vi "课堂.vi"() -> ()   [LabVIEW 2018]
panel:
  in  "停止 3":bool
  in  "等待时间（毫秒） 2":u32=1000
  out "布尔 4":bool
  out "布尔 3":bool
  out "布尔 2":bool
  out "平方根":dbl
  in  "数值":dbl
  out "数组 2":dbl[](array[numeric])
  in  "等待时间（毫秒）":u32
  in  "y 2":dbl
  in  "x 2":dbl
  in  "数组":enum16{"加法", "减法", "乘法", "除法", "清零"}[](array[ring])
  in  "停止 2":bool
  out "数值 3":dbl
  in  "y":dbl
  in  "x":dbl
  in  "枚举 2":enum16{"加法", "减法", "乘法", "除法", "清零"}(ring)
  in  "停止":bool
  out "字符串":string
  in  "枚举":enum16{"C", "B", "A"}(ring)
  out "x±1":dbl
  in  "x":dbl
  in  "布尔":bool
  # "灯亮x+1，灯灭x-1"
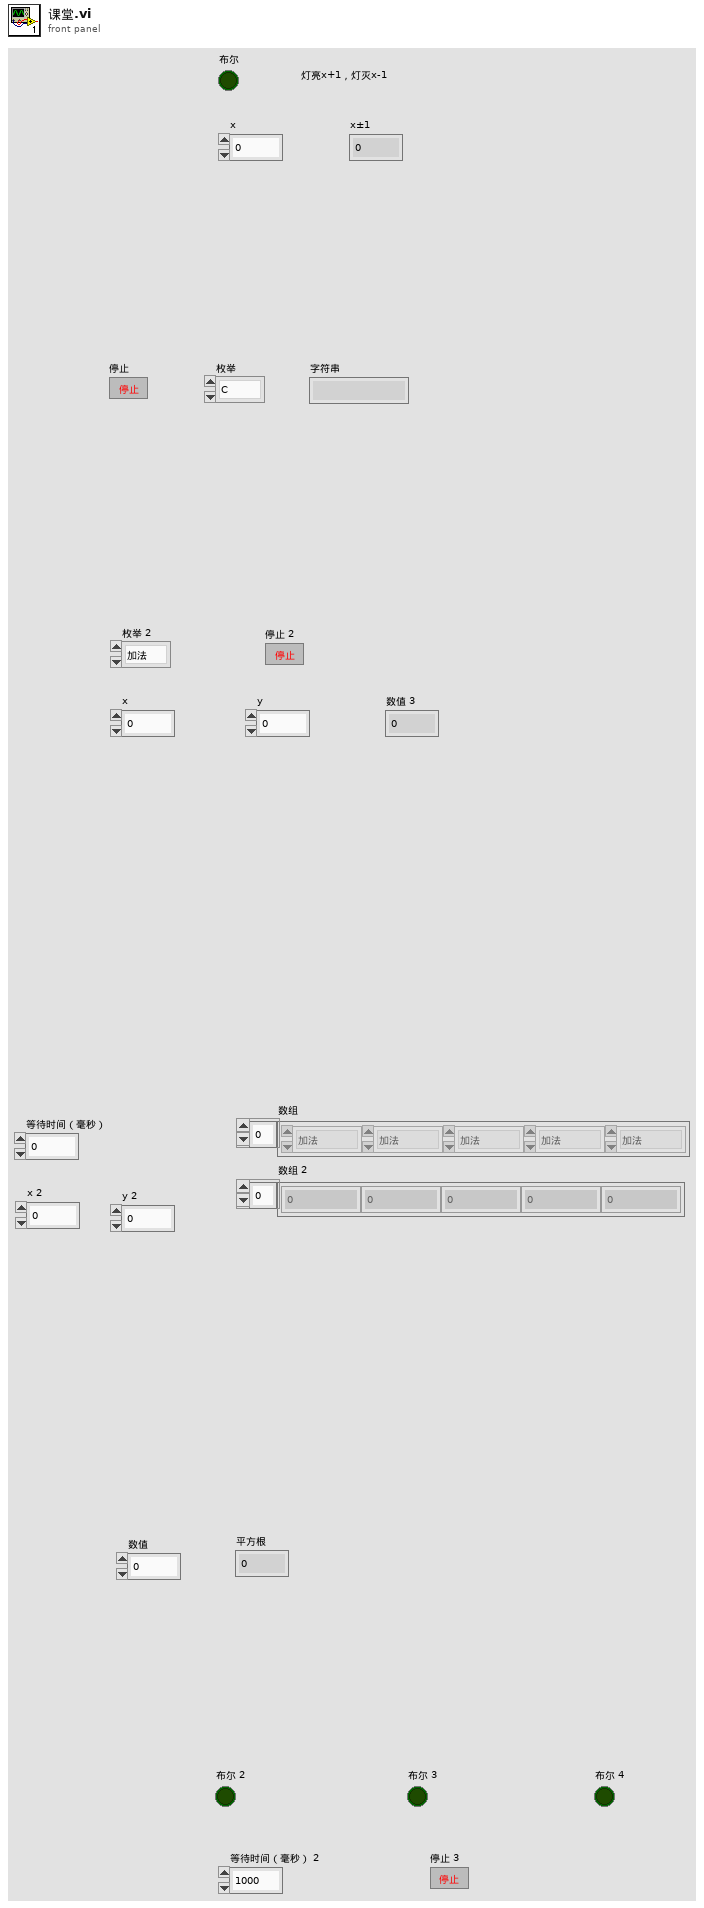
[diagram p1: front panel]
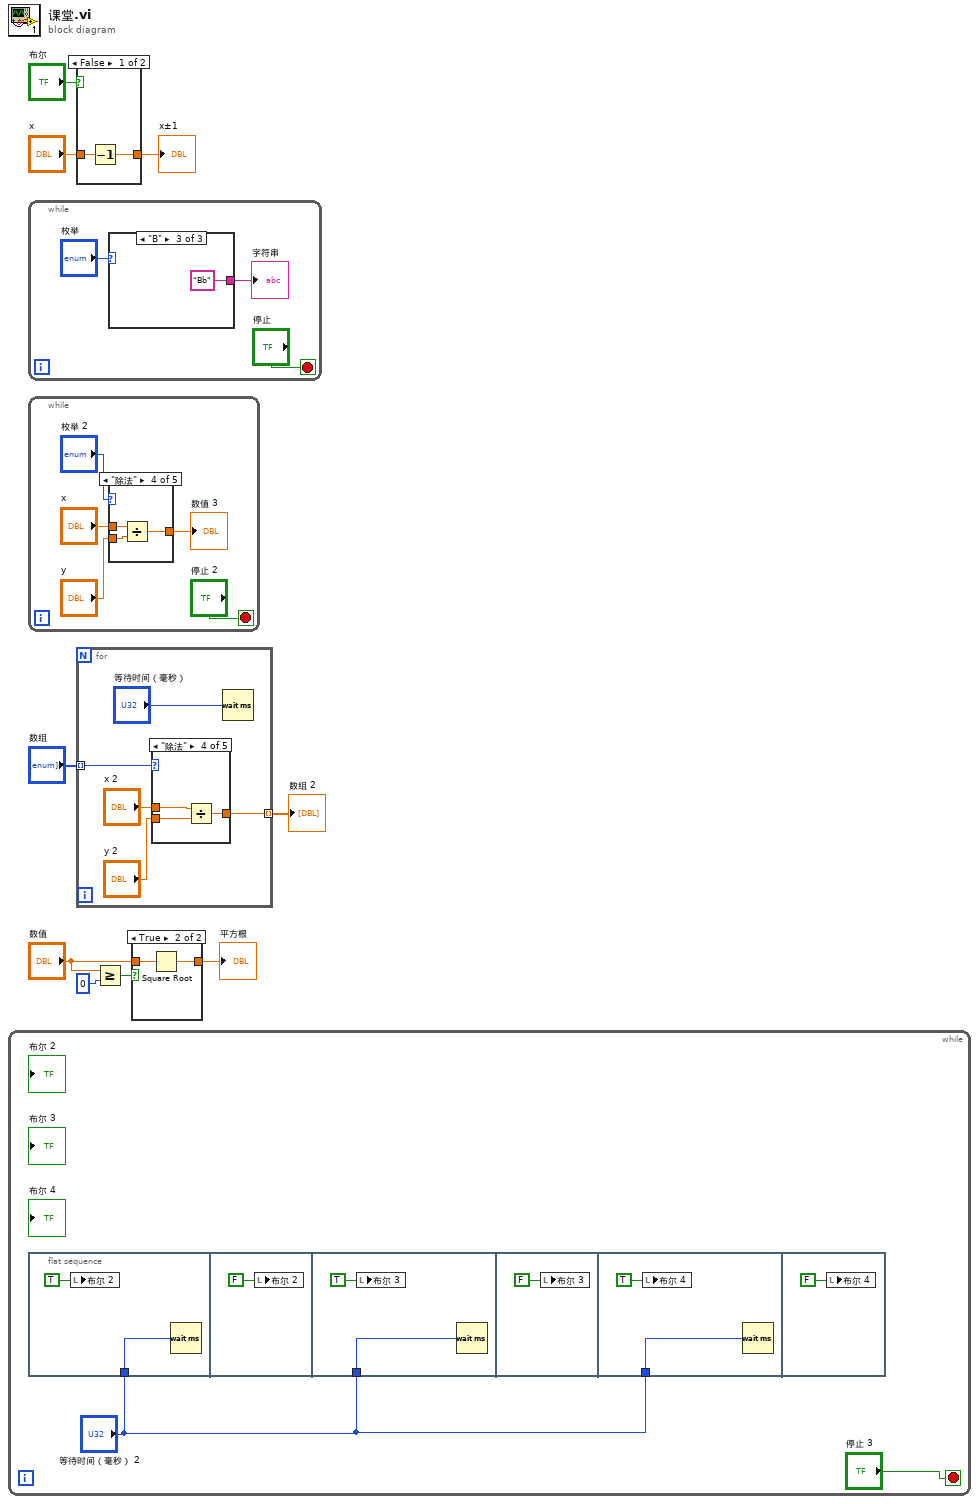
[diagram p0: block diagram]
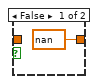
[diagram p2: hidden frame]
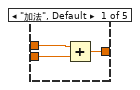
[diagram p3: hidden frame]
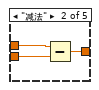
[diagram p4: hidden frame]
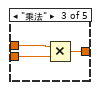
[diagram p5: hidden frame]
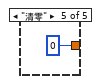
[diagram p6: hidden frame]
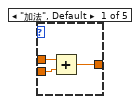
[diagram p7: hidden frame]
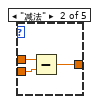
[diagram p8: hidden frame]
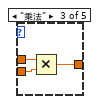
[diagram p9: hidden frame]
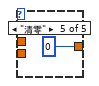
[diagram p10: hidden frame]
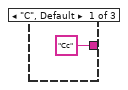
[diagram p11: hidden frame]
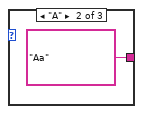
[diagram p12: hidden frame]
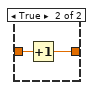
[diagram p13: hidden frame]
diagram:
  n1 = while {
    stop <- "停止 3" stop-if-true
    n2 = flat-sequence {
      tunnel: "等待时间（毫秒） 2" -> [w12]
      tunnel: "等待时间（毫秒） 2" -> [w15]
      tunnel: "等待时间（毫秒） 2" -> [w18]
      frame #0 {
        n3 = local write "布尔 2"(TRUE) -> ()
        n4 = Wait (ms)(milliseconds to wait=w12) -> ()  [unwired: 1 out]
      }
      frame #1 {
        n5 = local write "布尔 2"(FALSE) -> ()
      }
      frame #2 {
        n6 = local write "布尔 3"(TRUE) -> ()
        n7 = Wait (ms)(milliseconds to wait=w15) -> ()  [unwired: 1 out]
      }
      frame #3 {
        n8 = local write "布尔 3"(FALSE) -> ()
      }
      frame #4 {
        n9 = local write "布尔 4"(TRUE) -> ()
        n10 = Wait (ms)(milliseconds to wait=w18) -> ()  [unwired: 1 out]
      }
      frame #5 {
        n11 = local write "布尔 4"(FALSE ("布尔 4")) -> ()
      }
    }
  }
  n12 = while {
    stop <- "停止" stop-if-true
    n13 = case shown="\"B\"" "枚举" {
      tunnel: ["Cc" "Aa" "Bb"] -> w22
      frame "C", Default {
      }
      frame "A" {
      }
      frame "B" {
      }
    }
    "字符串" <- w22
  }
  n14 = while {
    stop <- "停止 2" stop-if-true
    n15 = case shown="\"除法\"" "枚举 2" {
      tunnel: "x" -> [w34 w37 w40 w43 _]
      tunnel: "y" -> [w33 w36 w39 w42 _]
      tunnel: [w32 w35 w38 w41 0] -> w28
      frame "加法", Default {
        n16 = Add(x=w34, y=w33) -> (x+y=w32:dbl)
      }
      frame "减法" {
        n17 = Subtract(x=w37, y=w36) -> (x-y=w35:dbl)
      }
      frame "乘法" {
        n18 = Multiply(x=w40, y=w39) -> (x*y=w38:dbl)
      }
      frame "除法" {
        n19 = Divide(x=w43, y=w42) -> (x/y=w41:dbl)
      }
      frame "清零" {
      }
    }
    "数值 3" <- w28
  }
  n20 = case shown="False" "布尔" {
    tunnel: "x" -> [w46 w48]
    tunnel: [w45 w47] -> w7
    frame False {
      n21 = Decrement(x=w46) -> (x-1=w45:dbl)
    }
    frame True {
      n22 = Increment(x=w48) -> (x+1=w47:dbl)
    }
  }
  "x±1" <- w7
  n23 = for {
    tunnel: "数组" -> [w51] mode=indexing
    tunnel: [w49] -> w5 mode=indexing
    n24 = case shown="\"除法\"" w51 {
      tunnel: "x 2" -> [w56 w59 w62 w65 _]
      tunnel: "y 2" -> [w55 w58 w61 w64 _]
      tunnel: [w54 w57 w60 w63 0] -> w49
      frame "加法", Default {
        n25 = Add(x=w56, y=w55) -> (x+y=w54:dbl)
      }
      frame "减法" {
        n26 = Subtract(x=w59, y=w58) -> (x-y=w57:dbl)
      }
      frame "乘法" {
        n27 = Multiply(x=w62, y=w61) -> (x*y=w60:dbl)
      }
      frame "除法" {
        n28 = Divide(x=w65, y=w64) -> (x/y=w63:dbl)
      }
      frame "清零" {
      }
    }
    n29 = Wait (ms)(milliseconds to wait="等待时间（毫秒）") -> ()  [unwired: 1 out]
  }
  "数组 2" <- w5
  n30 = Greater Or Equal?(x="数值", y=0) -> (x >= y?=w4:bool)
  n31 = case shown="True" w4 {
    tunnel: "数值" -> [_ w69]
    tunnel: [nan w68] -> w1
    frame False {
    }
    frame True {
      n32 = Square Root(x=w69) -> (sqrt(x)=w68:dbl)
    }
  }
  "平方根" <- w1
